vi "Standalone Initialize.vi"(8 "error in (no error)":errorcluster, 9 "Event-Registrations In":T1, 10 "Event-References In":T2, 11 "Actor in":refnum<class "Actor.lvclass">) -> (0 "error out":errorcluster, 1 "Event-Registrations Out":T1, 2 "Event-References Out":T2, 3 "Actor out":refnum<class "Actor.lvclass">, 4 "Standalone":bool)   [LabVIEW 2018, in "Actor.lvclass"]
uses:
  Actor.lvclass
  Event-References.ctl
  Stop.ctl
  Launched.ctl
  Event-Registrations.ctl
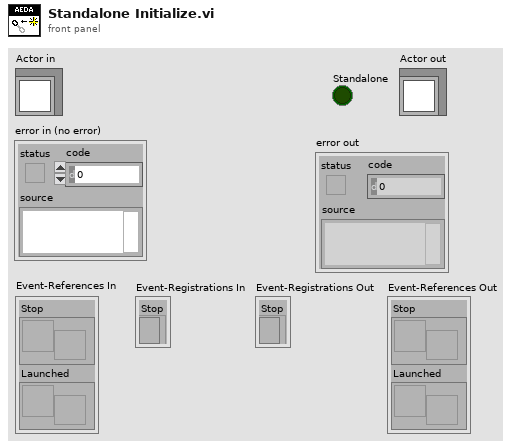
[diagram p1: front panel]
types:
  T1 = typedef "Actor.lvclass/Event-Registrations.ctl" = cluster{"Stop":refnum<event-registration>}
  T2 = typedef "Actor.lvclass/Event-References.ctl" = cluster{"Stop":refnum<user-event>, "Launched":refnum<user-event>}
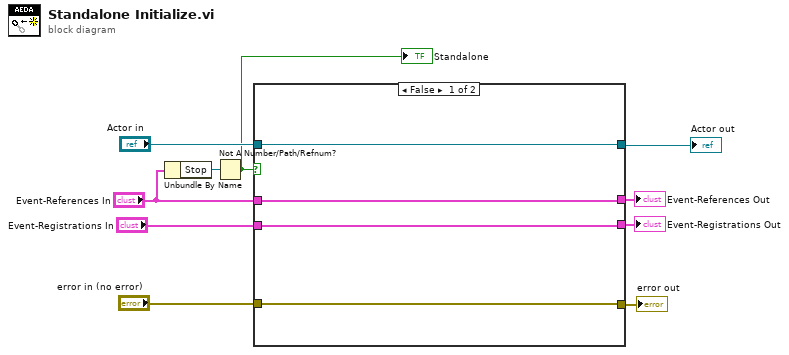
[diagram p0: block diagram]
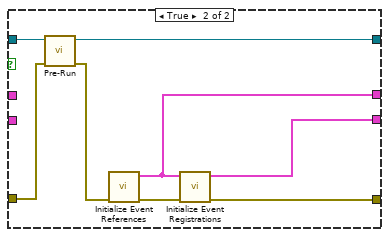
[diagram p2: hidden frame]
diagram:
  n1 = Unbundle By Name("Event-References In") -> ("Stop"=w9:refnum<user-event>)
  n2 = Not A Number/Path/Refnum?(number/path/refnum=w9) -> (NaN/Path/Refnum?=w7:bool)
  "Standalone" <- w7
  n3 = case shown="False" w7 {
    tunnel: "Actor in" -> [w14 w22]
    tunnel: "error in (no error)" -> [w12 w17]
    tunnel: "Event-References In" -> [w13 _]
    tunnel: [w12 w15] -> w5
    tunnel: [w13 w19] -> w3
    tunnel: [w14 w21] -> w4
    tunnel: [w11 w18] -> w2
    tunnel: "Event-Registrations In" -> [w11 _]
    frame False {
    }
    frame True {
      n4 = call-dynamic "Pre-Run.vi"("error in (no error)"=w17, "Actor in"=w22) -> ("error out"=w16:errorcluster, "Actor out"=w21:refnum<class "Actor.lvclass">)  [unwired: 8 in]
      n5 = call "Initialize Event References.vi"("error in (no error)"=w16) -> ("error out"=w20:errorcluster, "Event-References"=w19:T2)  [unwired: 9 in]
      n6 = call "Initialize Event Registrations.vi"("error in (no error)"=w20, "Events-References"=w19) -> ("error out"=w15:errorcluster, "Event-Registrations"=w18:T1)  [unwired: 8 in]
    }
  }
  "error out" <- w5
  "Actor out" <- w4
  "Event-References Out" <- w3
  "Event-Registrations Out" <- w2
